vi "lidarLines.vi"(7 "robotPosition":T1, 11 "points":cluster{dbl, dbl}[](array[cluster])) -> (0 "plots":cluster{sgl[], sgl[]}[](array[cluster]), 3 "segments":T2(array[cluster]))   [LabVIEW 2015]
uses:
  <vilib>/vision/NI_Vision_Development_Module.lvlib
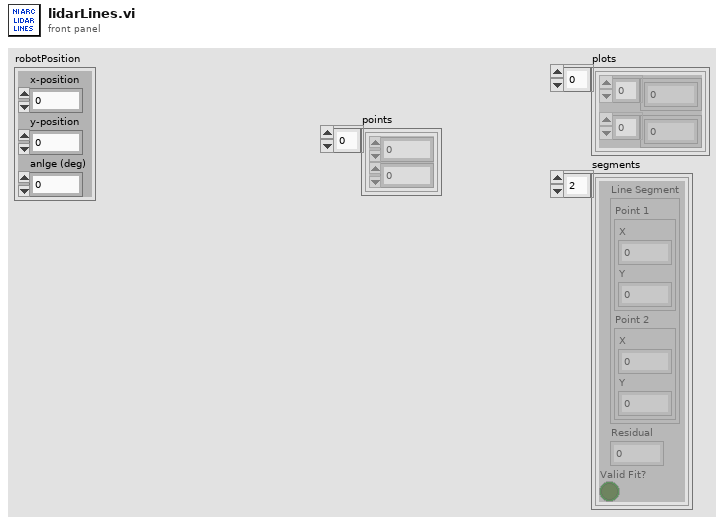
[diagram p1: front panel]
types:
  T1 = cluster{"x-position":dbl, "y-position":dbl, "anlge (deg)":dbl}
  T2 = cluster{"Line Segment":cluster{"Point 1":cluster{"X":sgl, "Y":sgl}, "Point 2":cluster{"X":sgl, "Y":sgl}}, "Residual":dbl, "Valid Fit?":bool}[]
  T3 = cluster{"Point 1":cluster{"X":sgl, "Y":sgl}, "Point 2":cluster{"X":sgl, "Y":sgl}}
  T4 = cluster{"Line Segment":cluster{"Point 1":cluster{"X":sgl, "Y":sgl}, "Point 2":cluster{"X":sgl, "Y":sgl}}, "Residual":dbl, "Valid Fit?":bool}
  T5 = cluster{"Line Segment":cluster{"Point 1":cluster{"X":sgl, "Y":sgl}, "Point 2":cluster{"X":sgl, "Y":sgl}}, "Residual":dbl, bool}
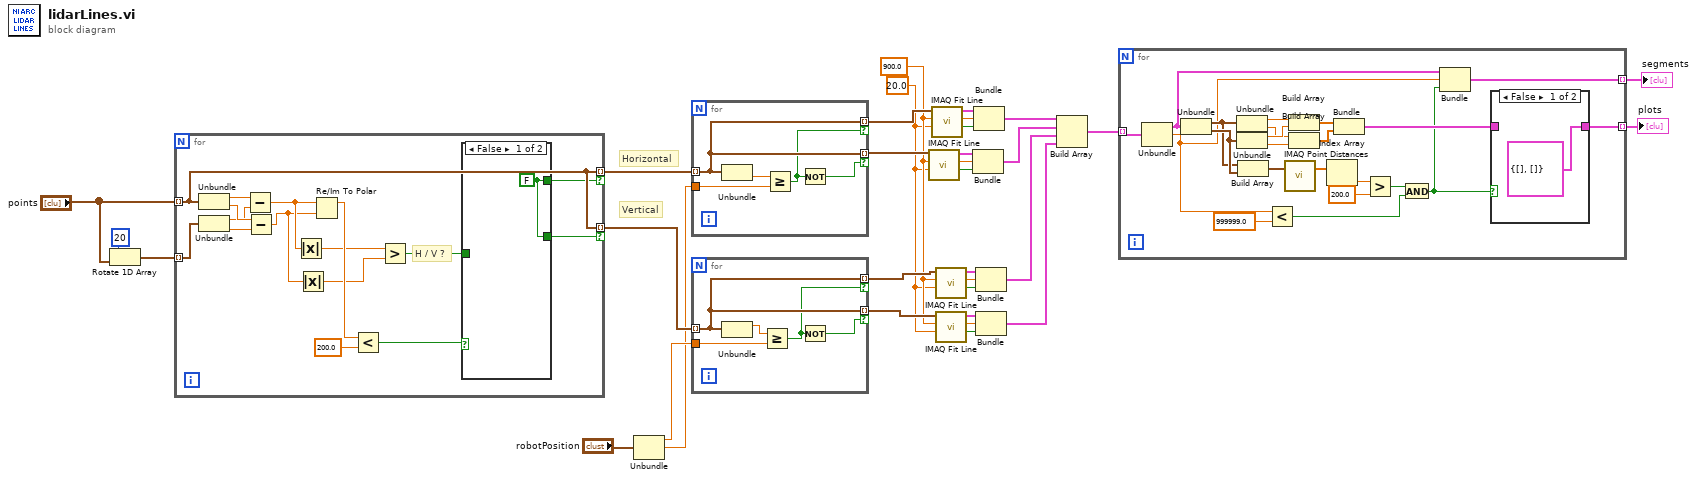
[diagram p0: block diagram]
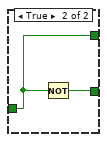
[diagram p3: hidden frame]
diagram:
  w24 = sgl 900.0 ("Minimum Score")
  w23 = sgl 20.0 ("Pixel Radius")
  # "Vertical"
  # "Horizontal"
  n1 = Rotate 1D Array(1:"points", 2:20 ("n")) -> (0:w32:cluster{dbl, dbl}[])
  n2 = for {
    tunnel: w32 -> [w43] mode=indexing
    tunnel: "points" -> [w38] mode=indexing
    tunnel: [w38] -> w31 mode=indexing if=w34
    tunnel: [w38] -> w30 mode=indexing if=w36
    # "H / V ?"
    n3 = Unbundle(w38) -> (w44:dbl, w46:dbl)
    n4 = Unbundle(w43) -> (w45:dbl, w47:dbl)
    n5 = Subtract(x=w44, y=w45) -> (x-y=w42:dbl)
    n6 = Subtract(x=w46, y=w47) -> (x-y=w41:dbl)
    n7 = Absolute Value(x=w42) -> (abs(x)=w40:dbl)
    n8 = Absolute Value(x=w41) -> (abs(x)=w39:dbl)
    n9 = Re/Im To Polar(2:w41, 3:w42) -> (1:w48:dbl)  [unwired: 1 out]
    n10 = Less?(x=w48, y=200.0) -> (x < y?=w37:bool)
    n11 = Greater?(x=w40, y=w39) -> (0:w35:bool)
    n12 = case shown="False" w37 {
      tunnel: [w50 w52] -> w36
      tunnel: w35 -> [_ w51]
      tunnel: [w50 w51] -> w34
      frame False {
        w50 = FALSE
      }
      frame True {
        n13 = Not(x=w51) -> (.not. x?=w52:bool)
      }
    }
  }
  n14 = Unbundle("robotPosition") -> ("x-position"=w2:dbl, "y-position"=w1:dbl)  [unwired: 1 out]
  n15 = for {
    tunnel: w31 -> [w57] mode=indexing
    tunnel: [w57] -> w26 mode=indexing if=w55
    tunnel: [w57] -> w29 mode=indexing if=w56
    tunnel: w1 -> [w53]
    n16 = Unbundle(w57) -> (w54:dbl)  [unwired: 1 out]
    n17 = Greater Or Equal?(x=w54, y=w53) -> (x >= y?=w55:bool)
    n18 = Not(x=w55) -> (.not. x?=w56:bool)
  }
  n19 = for {
    tunnel: w30 -> [w62] mode=indexing
    tunnel: [w62] -> w27 mode=indexing if=w60
    tunnel: [w62] -> w28 mode=indexing if=w61
    tunnel: w2 -> [w59]
    n20 = Unbundle(w62) -> (w58:dbl)  [unwired: 1 out]
    n21 = Greater Or Equal?(x=w58, y=w59) -> (x >= y?=w60:bool)
    n22 = Not(x=w60) -> (.not. x?=w61:bool)
  }
  n23 = call "IMAQ Fit Line"("Pixel Radius"=w23, "Minimum Score"=w24, "Points"=w29) -> ("Valid Fit?"=w17:bool, "Residual"=w18:dbl, "Line Segment"=w19:T3)  [unwired: 3 in, 3 out]
  n24 = call "IMAQ Fit Line"("Pixel Radius"=w23, "Minimum Score"=w24, "Points"=w26) -> ("Valid Fit?"=w20:bool, "Residual"=w21:dbl, "Line Segment"=w22:T3)  [unwired: 3 in, 3 out]
  n25 = call "IMAQ Fit Line"("Pixel Radius"=w23, "Minimum Score"=w24, "Points"=w27) -> ("Valid Fit?"=w14:bool, "Residual"=w15:dbl, "Line Segment"=w16:T3)  [unwired: 3 in, 3 out]
  n26 = call "IMAQ Fit Line"("Pixel Radius"=w23, "Minimum Score"=w24, "Points"=w28) -> ("Valid Fit?"=w11:bool, "Residual"=w12:dbl, "Line Segment"=w13:T3)  [unwired: 3 in, 3 out]
  n27 = Bundle("Line Segment"=w19, "Residual"=w18, "Valid Fit?"=w17) -> (w9:T4)  [unwired: 1 in]
  n28 = Bundle("Line Segment"=w22, "Residual"=w21, "Valid Fit?"=w20) -> (w10:T4)  [unwired: 1 in]
  n29 = Bundle("Line Segment"=w16, "Residual"=w15, "Valid Fit?"=w14) -> (w8:T4)  [unwired: 1 in]
  n30 = Bundle("Line Segment"=w13, "Residual"=w12, "Valid Fit?"=w11) -> (w7:T4)  [unwired: 1 in]
  n31 = Build Array(w10, w9, w8, w7) -> (w6:T2)
  n32 = for {
    tunnel: w6 -> [w84] mode=indexing
    tunnel: [w75] -> w5 mode=indexing
    tunnel: [w63] -> w4 mode=indexing
    n33 = Unbundle(w84) -> ("Line Segment"=w66:T3, "Residual"=w65:dbl)  [unwired: 1 out]
    n34 = Unbundle(w66) -> ("Point 1"=w72:cluster{"X":sgl, "Y":sgl}, "Point 2"=w73:cluster{"X":sgl, "Y":sgl})
    n35 = Unbundle(w72) -> ("X"=w83:sgl, "Y"=w81:sgl)
    n36 = Unbundle(w73) -> ("X"=w82:sgl, "Y"=w80:sgl)
    n37 = Build Array(w72, w73) -> (w74:cluster{"X":sgl, "Y":sgl}[])
    n38 = Less?(x=w65, y=999999.0) -> (x < y?=w67:bool)
    n39 = call "IMAQ Point Distances"("Points"=w74) -> ("Distances"=w71:sgl[])  [unwired: 4 in, 1 out]
    n40 = Build Array(w83, w82) -> (w79:sgl[])
    n41 = Build Array(w81, w80) -> (w78:sgl[])
    n42 = Index Array(array=w71) -> (element=w70:sgl)  [unwired: 1 in]
    n43 = Bundle(w79, w78) -> (w76:cluster{sgl[], sgl[]})  [unwired: 1 in]
    n44 = Greater?(x=w70, y=sgl 200.0) -> (0:w68:bool)
    n45 = And(x=w68, y=w67) -> (x .and. y?=w64:bool)
    n46 = Bundle("Line Segment"=w66, "Residual"=w65, w64) -> (w63:T5)  [unwired: 1 in]
    n47 = case shown="False" w64 {
      tunnel: w76 -> [_ w86]
      tunnel: [cluster{sgl[], sgl[]} {[], []} ("output cluster") w86] -> w75
      frame False {
      }
      frame True {
      }
    }
  }
  "plots" <- w5
  "segments" <- w4
